vi "LV Exp6.vi"   [LabVIEW 2009]
uses:
  <vilib>/NXT/Block Support/NXT_InputPort.ctl
  <vilib>/NXT/Dual Mode Library/Display/drawText.vi
  <vilib>/NXT/Dual Mode Library/Sensors/Read_Timer.vi
  <vilib>/NXT/Dual Mode Library/Sensors/Reset_Timer.vi
  <vilib>/NXT/Dual Mode Library/Waits/Wait_Num(msec).vi
panel:
  # "HiTechnic Experimenter's Kit\n\n                        Experiment 6 - Reaction Timer.\nThis program waits a random time, turns on the LED and measures how\nmuch time it takes for the red button to be pressed.\n\nSee Experimenter's Kit Handbook for the SuperPro for\nmore information or go to www.hitechnic.com\n\n(c) HiTechnic 2011"
types:
  T1 = typedef "NXT_InputPort.ctl" = u8
  T2 = typedef "LVHSConnector.ctl" = cluster{"error":errorcluster, "address":string, "NXT #":i32, "Show Error":bool, "Connection":u16}
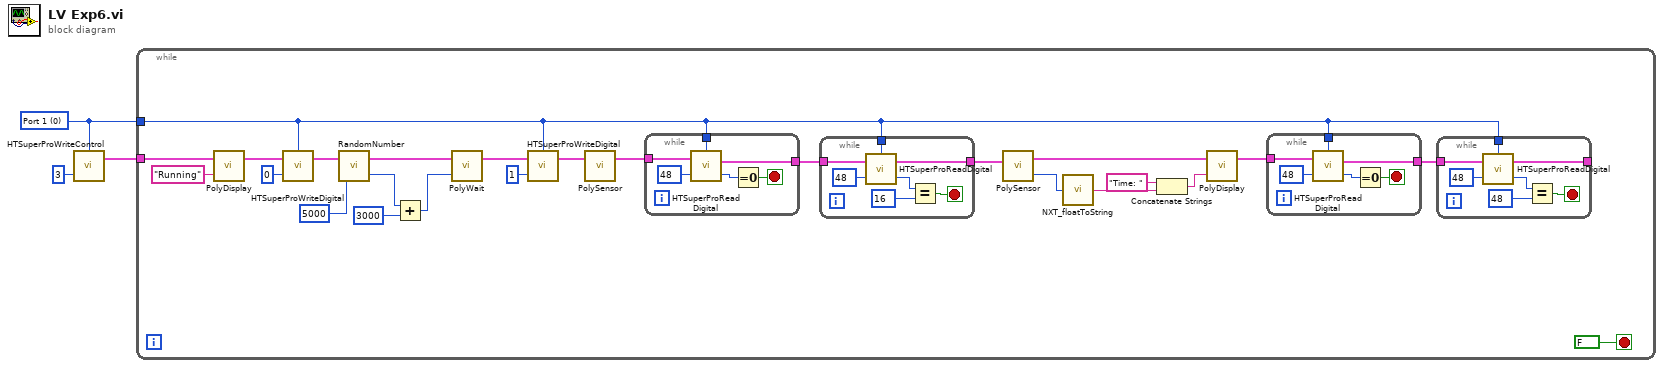
[diagram p0: block diagram]
diagram:
  w1 = T1 0 items=["Port 1", "Port 2", "Port 3", "Port 4"] ("Port")
  n1 = call "HTSuperProWriteControl.vi"("Digital Value"=u8 3, "Port"=w1) -> ("NXT"=w2:T2)  [unwired: 3 in]
  n2 = while {
    tunnel: w2 -> [w28]
    tunnel: w1 -> [w5]
    stop <- FALSE stop-if-true
    n3 = call-poly <vilib>:"PolyDisplay.vi"("Text"="Running", "NXT"=w28) -> ("NXT"=w26:T2)  [unwired: 2 in]
    n4 = call "HTSuperProWriteDigital.vi"("Digital Value"=u8 0, "NXT"=w26, "Port"=w5) -> ("NXT"=w24:T2)  [unwired: 2 in]
    n5 = call <vilib>:"RandomNumber.vi"("Max Value"=i16 5000, "NXT"=w24) -> ("Random Number"=w22:u16, "NXT"=w20:T2)  [unwired: 1 in]
    n6 = Add(x=w22, y=i16 3000) -> (x+y=w19:u16)
    n7 = call-poly <vilib>:"PolyWait.vi"("Time (100 msec)"=w19, "NXT"=w20) -> ("NXT"=w17:T2)  [unwired: 2 in]
    n8 = call "HTSuperProWriteDigital.vi"("Digital Value"=u8 1, "NXT"=w17, "Port"=w5) -> ("NXT"=w15:T2)  [unwired: 2 in]
    n9 = call-poly <vilib>:"PolySensor.vi"("NXT"=w15) -> ("NXT"=w14:T2)  [unwired: 3 in]
    n10 = while {
      tunnel: w14 -> [w54]
      tunnel: w5 -> [w50]
      tunnel: [w49] -> w16
      stop <- w51 stop-if-true
      n11 = call "HTSuperProReadDigital.vi"("Mask"=u8 48, "NXT"=w54, "Port"=w50) -> ("Digital Value"=w52:u8, "NXT"=w49:T2)  [unwired: 1 in]
      n12 = Equal To 0?(x=w52) -> (x = 0?=w51:bool)
    }
    n13 = while {
      tunnel: w16 -> [w48]
      tunnel: w5 -> [w43]
      tunnel: [w42] -> w13
      stop <- w44 stop-if-true
      n14 = call "HTSuperProReadDigital.vi"("Mask"=u8 48, "NXT"=w48, "Port"=w43) -> ("Digital Value"=w46:u8, "NXT"=w42:T2)  [unwired: 1 in]
      n15 = Equal?(x=w46, y=u8 16 ("Mask")) -> (x = y?=w44:bool)
    }
    n16 = call-poly <vilib>:"PolySensor.vi"("NXT"=w13) -> ("Value (msec)"=w10:u32, "NXT"=w12:T2)  [unwired: 2 in]
    n17 = call <vilib>:"NXT_floatToString.vi"("number"=w10) -> ("string"=w9:string)
    n18 = Concatenate Strings("Time: " ("string"), w9) -> (w11:string)
    n19 = call-poly <vilib>:"PolyDisplay.vi"("Text"=w11, "NXT"=w12) -> ("NXT"=w7:T2)  [unwired: 2 in]
    n20 = while {
      tunnel: w7 -> [w41]
      tunnel: w5 -> [w37]
      tunnel: [w36] -> w6
      stop <- w38 stop-if-true
      n21 = call "HTSuperProReadDigital.vi"("Mask"=u8 48, "NXT"=w41, "Port"=w37) -> ("Digital Value"=w39:u8, "NXT"=w36:T2)  [unwired: 1 in]
      n22 = Equal To 0?(x=w39) -> (x = 0?=w38:bool)
    }
    n23 = while {
      tunnel: w6 -> [w35]
      tunnel: w5 -> [w30]
      tunnel: [w29] -> _
      stop <- w31 stop-if-true
      n24 = call "HTSuperProReadDigital.vi"("Mask"=u8 48, "NXT"=w35, "Port"=w30) -> ("Digital Value"=w33:u8, "NXT"=w29:T2)  [unwired: 1 in]
      n25 = Equal?(x=w33, y=u8 48 ("Mask")) -> (x = y?=w31:bool)
    }
  }
